vi "Read Device State.vi"(8 "Error In":errorcluster, 11 "AMS Connection In":T2) -> (0 "Error Out":errorcluster, 2 "Device State":u16, 3 "ADS State":T1)   [LabVIEW 2016, in "TwinCAT ADS.lvlib"]
uses:
  TwinCAT ADS.lvlib
  Low Level/TypeDefs/AMS Connection.ctl
  Low Level/TypeDefs/AMS.ctl
  Low Level/TypeDefs/ADS States.ctl
  Low Level/TypeDefs/Command Id.ctl
  Low Level/TypeDefs/State Flag.ctl
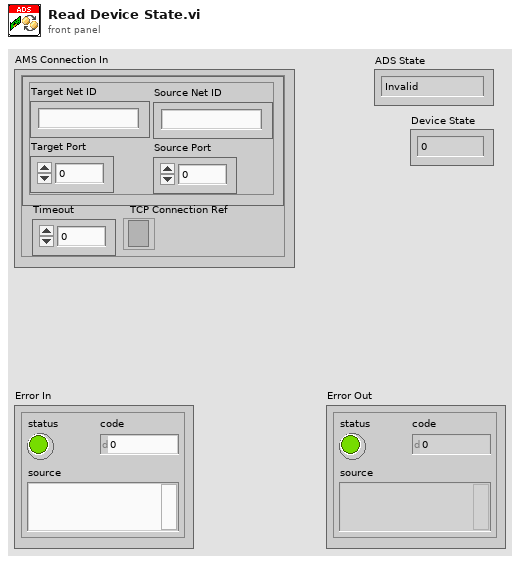
[diagram p1: front panel]
types:
  T1 = typedef "TwinCAT ADS.lvlib/ADS States.ctl" = enum16{"Invalid", "Idle", "Reset", "Init", "Start", "Run", "Stop", "SaveCfg", "LoadCfg", "PowerFailure", "PowerGood", "Error", "Shutdown", "Suspend", "Resume", "Config", "Reconfig"}
  T2 = typedef "TwinCAT ADS.lvlib/AMS Connection.ctl" = cluster{"AMS":T3, "Timeout":i32, "TCP Connection Ref":refnum<k5>}
  T3 = typedef "TwinCAT ADS.lvlib/AMS.ctl" = cluster{"Target Net ID":string, "Target Port":u16, "Source Net ID":string, "Source Port":u16}
  T4 = enum16{"Standard", "Buffered", "CRLF", "Immediate"}
  T5 = typedef "TwinCAT ADS.lvlib/State Flag.ctl" = u16
  T6 = typedef "TwinCAT ADS.lvlib/Command Id.ctl" = enum16{"Invalid", "ADS Read Device Info", "ADS Read", "ADS Write", "ADS Read State", "ADS Write Control", "ADS Add Device Notification", "ADS Delete Device Notification", "ADS Device Notification", "ADS Read Write"}
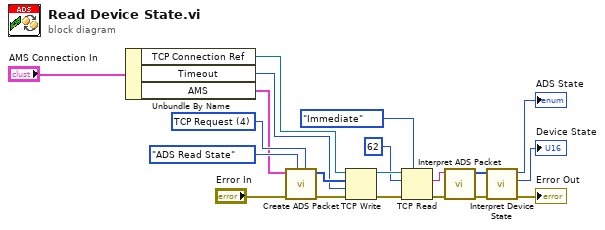
[diagram p0: block diagram]
diagram:
  w19 = T5 4 items=["TCP Request"=4, "TCP Response"=5, "UDP Request"=68, "UDP Respone"=69] ("State Flag")
  n1 = Unbundle By Name("AMS Connection In") -> ("TCP Connection Ref"=w3:refnum<k5>, "Timeout"=w2:i32, "AMS"=w4:T3)
  n2 = call "Create ADS Packet.vi"("State Flag"=w19, "Command ID"=Command_Id."ADS Read State", "Error In"="Error In", "AMS"=w4) -> ("Error Out"=w16:errorcluster, "ADS Packet"=w18:u8[])  [unwired: 6 in]
  n3 = TCP Write(connection ID=w3, data in=w18, error in (no error)=w16, 9:w2) -> (connection ID out=w17:refnum<k5>, error out=w15:errorcluster)  [unwired: 1 out]
  n4 = TCP Read(connection ID=w17, bytes to read=62, error in (no error)=w15, 7:T4."Immediate" ("mode (standard)")) -> (data out=w10:string, error out=w11:errorcluster)  [unwired: 1 in, 1 out]
  n5 = call "Interpret ADS Packet.vi"("Error In"=w11, "ADS Packet"=w10) -> ("Error Out"=w8:errorcluster, "Data"=w9:u8[])  [unwired: 3 in, 5 out]
  n6 = call "Interpret Device State.vi"("Error In"=w8, "Data In"=w9) -> ("Error Out"=→"Error Out":errorcluster, "Device State"=→"Device State":u16, "ADS State"=→"ADS State":T1)  [unwired: 6 in, 1 out]
